vi "十進制傳PLC.vi"(7 "位數":i32=9, 8 "error in (no error)":errorcluster, 9 "input string":string, 10 "PLC address":i32=20, 11 "Input Data":i32=222) -> (0 "error out":errorcluster, 3 "Array":u16[](array[numeric]))   [LabVIEW 2019]
uses:
  Ctrl/ModbusCmd.ctl
panel:
  in  "array":u16[](array[numeric])
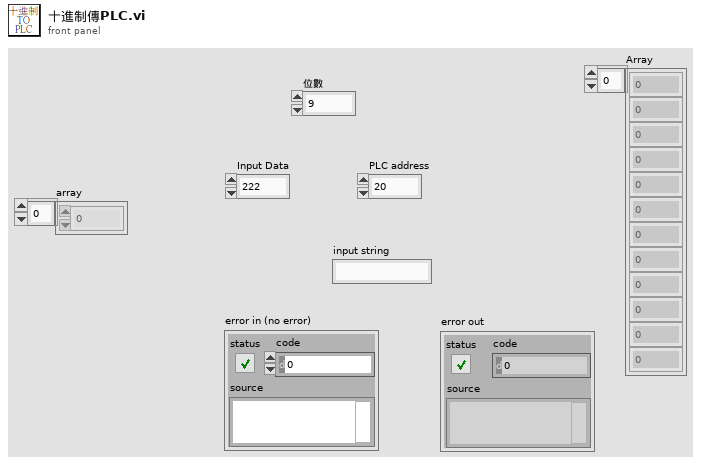
[diagram p1: front panel]
types:
  T1 = cluster{"starting address":u16, "number of inputs":u16, "Sat Coils":bool[], "Holding Registers":u16[]}
  T2 = typedef "ModbusCmd.ctl" = enum16{"Connect", "Disconnect", "Init", "Fetch Basic Objects", "Fetch Input Refisters", "Fetch Discrete Inputs", "Set Coils", "Set Holding Registers", "Write Single Holding", "Exit"}
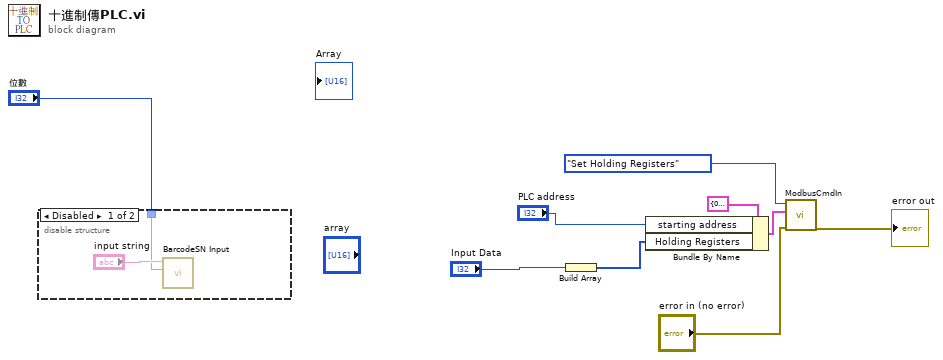
[diagram p0: block diagram]
diagram:
  n1 = disable-structure shown="Disabled" {
    disable-tunnel: "位數" -> [w10 _]
    frame Disabled {
      n2 = call "BarcodeSN Input.vi"("位數"=w10, "String Input"="input string") -> ()  [unwired: 9 in, 1 out]
    }
    frame Enabled {
    }
  }
  n3 = Build Array("Input Data") -> (w3:i32[])
  n4 = Bundle By Name(cluster=T1 {"starting address"=0, "number of inputs"=0, "Sat Coils"=[FALSE], "Holding Registers"=[]} ("data"), "starting address"="PLC address", "Holding Registers"=w3) -> (w6:T1)
  n5 = call "ModbusCmdIn.vi"("error in (no error)"="error in (no error)", "data"=w6, "Enum"=ModbusCmd."Set Holding Registers") -> ("error out"=→"error out":errorcluster)  [unwired: 8 in]
